vi "SW_Get_CPU_load.vi"(4 "error in (no error)":errorcluster, 5 "Buffer length, sec":dbl=5.0 min=0.1 max=120.0 step=0.1, 6 "Scan interval, ms":u32=250 min=25 max=5000 step=25, 7 "CPU monitor .NET reference in":refnum<k24>) -> (0 "error out":errorcluster, 1 "Historical CPU load, %":sgl format="%_6g", 2 "Instant CPU load, %":sgl format="%_6g", 3 "CPU monitor .NET reference out":refnum<k24>)   [LabVIEW 2018, in "Tracker.lvlib"]
uses:
  Tracker.lvlib
  <vilib>/Analysis/baseanly.llb/Mean (DBL).vi
  Common_Resources.lvlib
  <vilib>/Analysis/NI_AALBase.lvlib
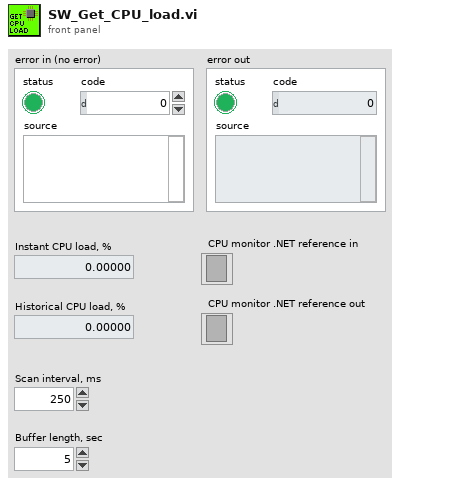
[diagram p1: front panel]
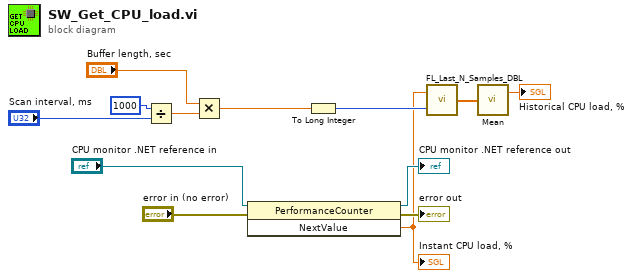
[diagram p0: block diagram]
diagram:
  n1 = Divide(x=u32 1000, y="Scan interval, ms") -> (x/y=w8:dbl)
  n2 = Multiply(x="Buffer length, sec", y=w8) -> (x*y=w9:dbl)
  n3 = invoke class="PerformanceCounter" method="NextValue"(reference="CPU monitor .NET reference in", error in="error in (no error)") -> (reference out=→"CPU monitor .NET reference out":refnum<k24>, error out=→"error out":errorcluster, "NextValue"=w3:sgl)  [unwired: 1 in]
  "Instant CPU load, %" <- w3
  n4 = To Long Integer(number=w9) -> (32bit integer=w4:i32)
  n5 = call "FL_Last_N_Samples_DBL.vi"("BufferLengthSamples"=w4, "Input sample"=w3) -> ("Output Array"=w6:dbl[])
  n6 = call-poly <vilib>:"Mean.vi"("X"=w6) -> ("mean"=→"Historical CPU load, %":dbl)  [unwired: 1 out]
